vi "CreatePublicEvents.vi"(8 "error in (no error)":errorcluster, 11 "Generator":refnum<class "Generator.lvclass">) -> (0 "error out":errorcluster, 3 "Generator out":refnum<class "Generator.lvclass">)   [LabVIEW 2019, in "Generator.lvclass"]
uses:
  Generator.lvclass
  <vilib>/JKI/JKI SMO/SMO/SMO.lvclass
panel:
  # "For instructions on how to use the JKI State Machine Objects, examples and video tutorials, visit:\nhttp://jki.net/state-machine-objects/\n\nJKI State Machine Objects™\nhttp://jki.net/state-machine-objects/\nCopyright (C) 2005-2015, JKI <info@jki.net>\nALL RIGHTS RESERVED"
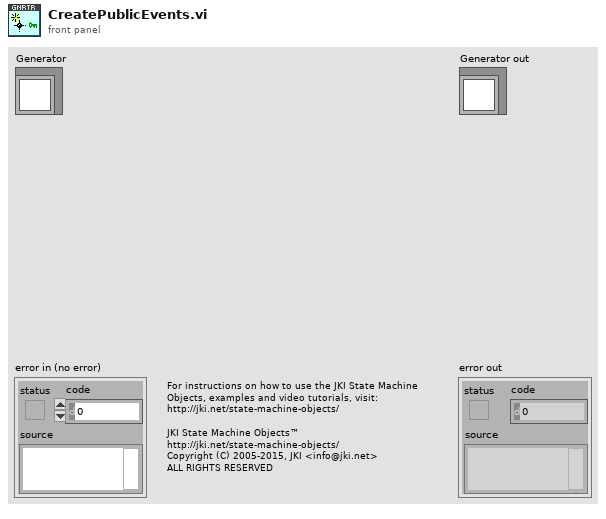
[diagram p1: front panel]
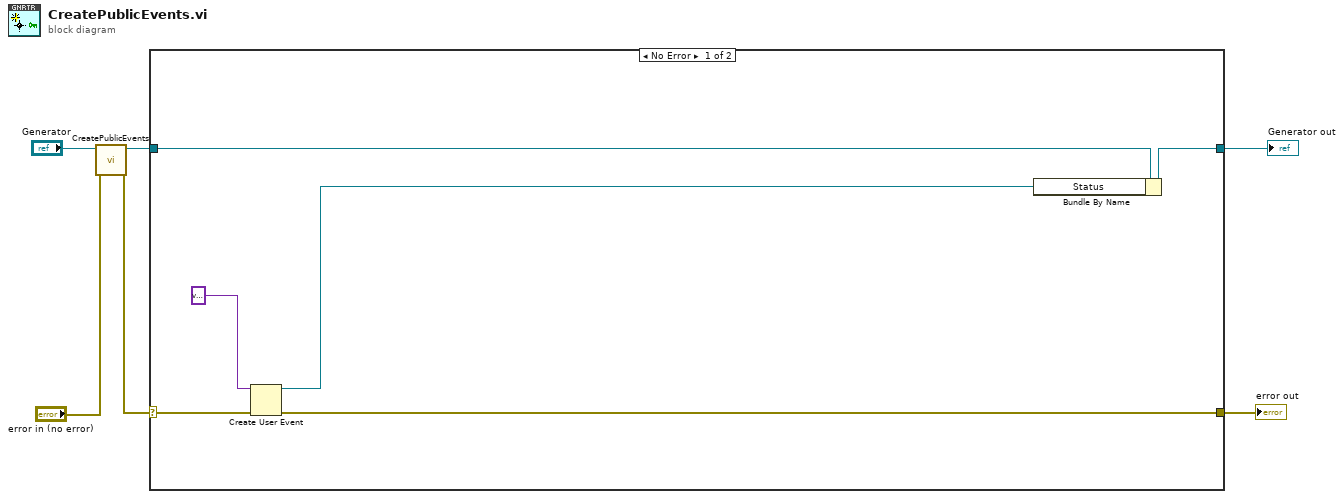
[diagram p0: block diagram]
diagram:
  n1 = call-parent "CreatePublicEvents.vi"("error in (no error)"="error in (no error)", "SMO"="Generator") -> ("error out"=w1:errorcluster, "SMO out"=w5:refnum<class "Generator.lvclass">)  [unwired: 8 in]
  n2 = case shown="No Error" w1 {
    selector: w1 -> [w11 w14]
    tunnel: [w8 w14] -> w3
    tunnel: [w12 w13] -> w4
    tunnel: w5 -> [w9 w13]
    frame No Error {
      n3 = Create User Event(user event datatype=variant, error in=w11) -> (user event=w10:refnum<user-event>, error out=w8:errorcluster)
      n4 = Bundle By Name(cluster=w9, "Status"=w10) -> (w12:refnum<class "Generator.lvclass">)
    }
    frame Error {
    }
  }
  "error out" <- w3
  "Generator out" <- w4
